vi "FPGA Main NoStartEnc.vi"() -> ()   [LabVIEW 2009]
uses:
  <vilib>/Platform/TimedLoop/XDataNode/XDataNode.xnode
  <vilib>/Platform/TimedLoop/XDataNode/loadlvalarms.vi
  <vilib>/Platform/TimedLoop/XDataNode/timing_clust.ctl
  <vilib>/Platform/TimedLoop/XDataNode/nitl_modes.ctl
  <vilib>/Platform/TimedLoop/XDataNode/wakeup.ctl
  <vilib>/eio/EIONode/EIONode.xnode
  <vilib>/rvi/eio/nirviEIOImplementation/nirviEIOImplementation.xnode
  <vilib>/rvi/eio/common/nirviEmuTemplateMethod_noerrors.vi
  <vilib>/rvi/eio/common/nirviEmuClasses.ctl
  <vilib>/Platform/TimedLoop/XDataNode/XDNodeRunTimeDep.lvlib
  <vilib>/NI VeriStand/FPGA/NI_VS FPGA Support.lvlib
panel:
  out "Travel dT (Ticks)":u32
  out "Pitch dT (Ticks)":u32
  out "Elevation dT (Ticks)":u32
  out "Travel Set High":u32
  in  "Clock Divider":u16=500
  out "Reset?":bool
  out "Travel Velocity":i32
  out "Travel Position":i32
  out "ENC 2 In Vel/Acc Update":bool
  out "Pitch Velocity":i32
  out "Pitch Position":i32
  out "ENC 1 In Vel/Acc Update":bool
  out "Elevation Velocity":i32
  out "Elevation Position":i32
  out "ENC 0 In Vel/Acc Update":bool
  in  "ENC In Clock":bool=TRUE
  in  "Fan High Time 2":u32
  in  "Fan High Time 1":u32
  out "Elevation Set High":u32
  in  "PWM Period (ticks)":u32=100000
  # "PWM In"
  # "Configuration"
  # "Internal Controls"
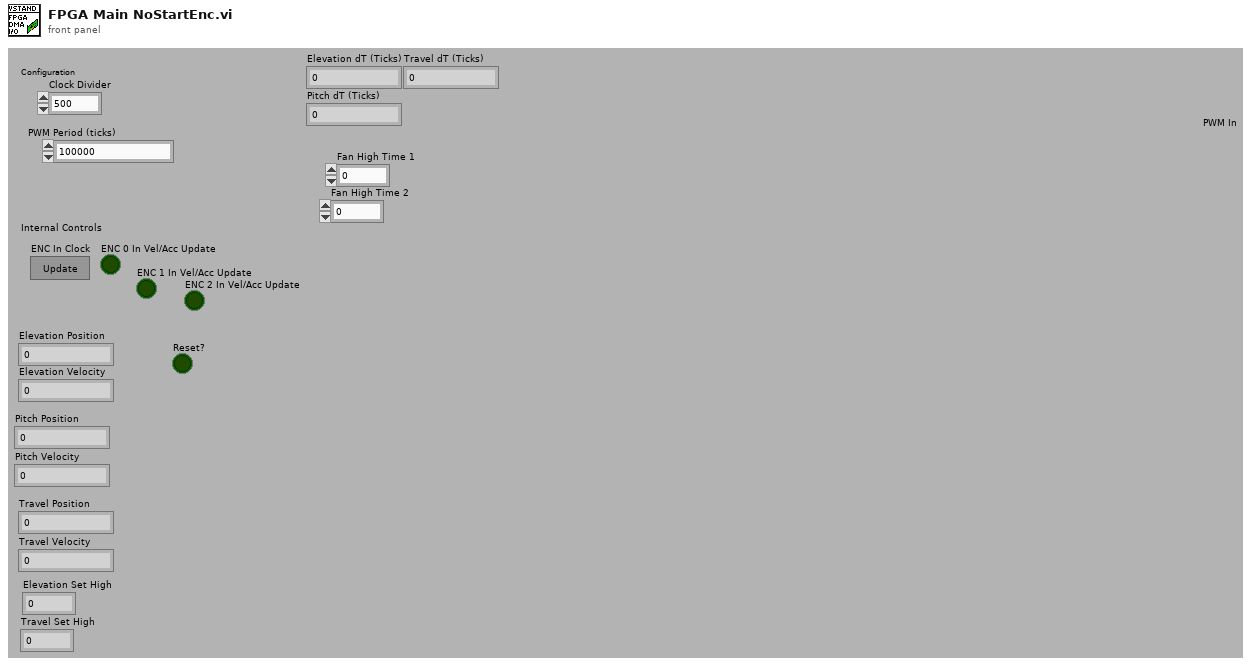
[diagram p1: front panel]
types:
  T1 = typedef "XDNodeRunTimeDep.lvlib/timing_clust.ctl" = cluster{"Expected End [f-1]":u64, "Actual End [f-1]":u64, "Finished Late? [f-1]":bool, "Expected End [i-1]":u64, "Actual End [i-1]":u64, "Finished Late? [i-1]":bool, "Expected Start [i]":u64, "Actual Start [i]":u64, "Expected Start [f]":u64, "Actual Start [f]":u64, "Source Name":string, "Structure Name":string, "Period":i64, "Deadline":i64, "Offset":i64, "Start":i64, "Priority":i32, "Timeout":i32, "Mode":T2, "Wakeup Reason":T3, "Error":errorcluster, "Source Type":string, "Secondary Source Type":string, "Global End Time":u64, "Global Start Time":u64, "Frame Duration":u64, "Iteration Duration":u64, "Assigned CPU":i32, "I/O Scan Engine Mode":u32}
  T2 = typedef "XDNodeRunTimeDep.lvlib/nitl_modes.ctl" = enum32{"No Change", "Process missed periods, maintain original phase", "Discard missed periods, maintain original phase", "Process missed periods, ignore original phase", "Discard missed periods, ignore original phase"}
  T3 = typedef "XDNodeRunTimeDep.lvlib/wakeup.ctl" = enum32{"Normal", "Aborted", "Asynchronous wakeup", "Timing source error", "Timed loop error", "Timeout"}
  T4 = typedef "nirviEmuClasses.ctl" = enum16{"IO Read", "IO Write", "Method", "Property Read", "Property Write"}
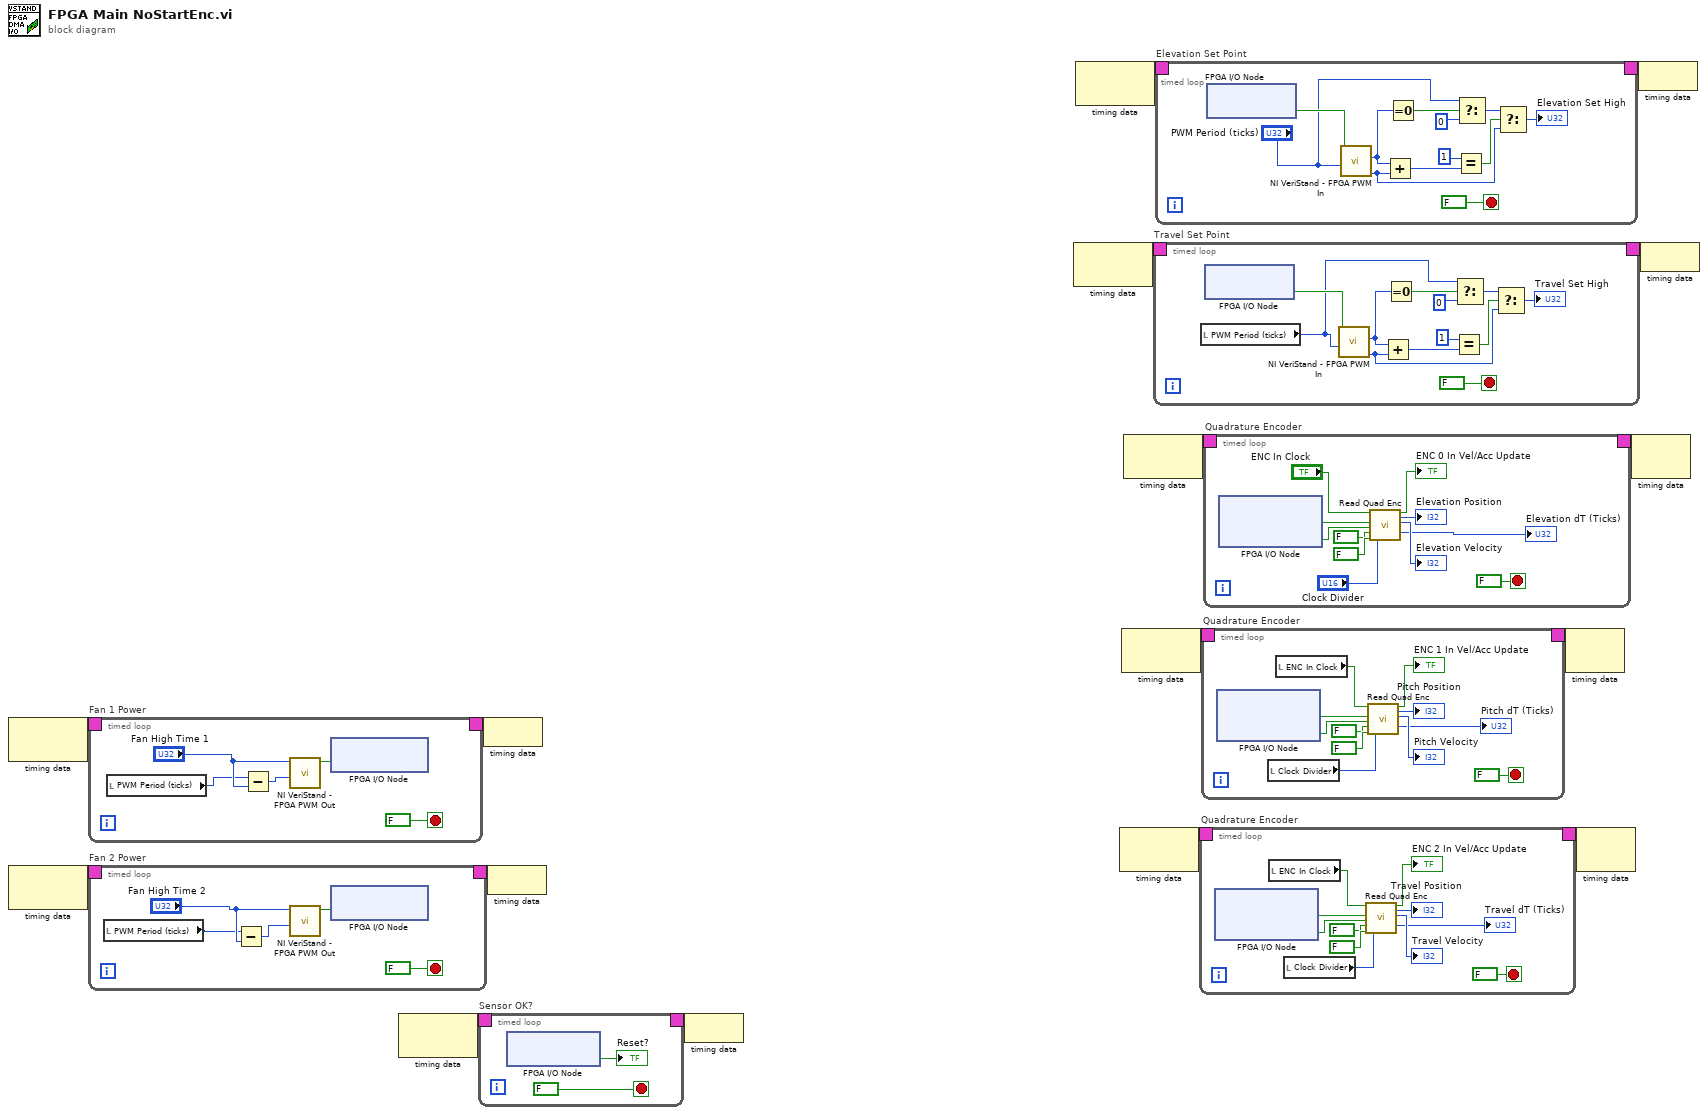
[diagram p0: block diagram]
diagram:
  n1 = node-c288() -> (w16:T1)  [unwired: 1 in]
  n2 = node-c288() -> (w14:T1)  [unwired: 1 in]
  n3 = timed-loop "Fan 1 Power" {
    timing: w16 -> [_]
    timing-out: [_] -> w15
    stop <- FALSE stop-if-true
    n4 = local read "PWM Period (ticks)"() -> (w17:u32)
    n5 = Subtract(x=w17, y="Fan High Time 1") -> (x-y=w19:u32)
    n6 = call <vilib>:"NI VeriStand - FPGA PWM Out.vi"("_Low Time"=w19, "_High Time"="Fan High Time 1") -> ("Output"=w20:bool)  [unwired: 9 in]
    n7 = xnode "FPGA I/O Node"("PWM 2 Out"=w20) -> ()  [unwired: 1 in, 1 out]
  }
  n8 = timed-loop "Fan 2 Power" {
    timing: w14 -> [_]
    timing-out: [_] -> w13
    stop <- FALSE stop-if-true
    n9 = local read "PWM Period (ticks)"() -> (w35:u32)
    n10 = Subtract(x=w35, y="Fan High Time 2") -> (x-y=w36:u32)
    n11 = call <vilib>:"NI VeriStand - FPGA PWM Out.vi"("_Low Time"=w36, "_High Time"="Fan High Time 2") -> ("Output"=w38:bool)  [unwired: 9 in]
    n12 = xnode "FPGA I/O Node"("PWM 3 Out"=w38) -> ()  [unwired: 1 in, 1 out]
  }
  n13 = node-c288() -> (w12:T1)  [unwired: 1 in]
  n14 = timed-loop "Sensor OK?" {
    timing: w12 -> [_]
    timing-out: [_] -> w11
    stop <- FALSE stop-if-true
    n15 = xnode "FPGA I/O Node"() -> ("Sensor OK"=→"Reset?":bool)  [unwired: 1 in, 1 out]
  }
  n16 = node-c288(w15) -> ()
  n17 = node-c288(w13) -> ()
  n18 = node-c288(w11) -> ()
  n19 = node-c288() -> (w2:T1)  [unwired: 1 in]
  n20 = node-c288() -> (w10:T1)  [unwired: 1 in]
  n21 = node-c288() -> (w4:T1)  [unwired: 1 in]
  n22 = node-c288() -> (w6:T1)  [unwired: 1 in]
  n23 = node-c288() -> (w8:T1)  [unwired: 1 in]
  n24 = timed-loop "Travel Set Point" {
    timing: w2 -> [_]
    timing-out: [_] -> w1
    stop <- FALSE stop-if-true
    n25 = local read "PWM Period (ticks)"() -> (w76:u32)
    n26 = xnode "FPGA I/O Node"() -> ("PWM 1 In"=w86:bool)  [unwired: 1 in, 1 out]
    n27 = call <vilib>:"NI VeriStand - FPGA PWM In.vi"("Time Out"=w76, "Value"=w86) -> ("High time"=w82:u32, "Low Time"=w80:u32)  [unwired: 8 in]
    n28 = Add(x=w80, y=w82) -> (x+y=w85:u32)
    n29 = Equal To 0?(x=w80) -> (x = 0?=w81:bool)
    n30 = Equal?(x=u32 1, y=w85) -> (x = y?=w83:bool)
    n31 = Select(t=w76, s=w81, f=u32 0) -> (s? t:f=w78:u32)
    n32 = Select(t=w78, s=w83, f=w82) -> (s? t:f=→"Travel Set High":u32)
  }
  n33 = timed-loop "Elevation Set Point" {
    timing: w10 -> [_]
    timing-out: [_] -> w9
    stop <- FALSE stop-if-true
    n34 = xnode "FPGA I/O Node"() -> ("PWM 0 In"=w119:bool)  [unwired: 1 in, 1 out]
    n35 = call <vilib>:"NI VeriStand - FPGA PWM In.vi"("Time Out"="PWM Period (ticks)", "Value"=w119) -> ("High time"=w115:u32, "Low Time"=w113:u32)  [unwired: 8 in]
    n36 = Add(x=w113, y=w115) -> (x+y=w118:u32)
    n37 = Equal To 0?(x=w113) -> (x = 0?=w114:bool)
    n38 = Equal?(x=u32 1, y=w118) -> (x = y?=w116:bool)
    n39 = Select(t="PWM Period (ticks)", s=w114, f=u32 0) -> (s? t:f=w111:u32)
    n40 = Select(t=w111, s=w116, f=w115) -> (s? t:f=→"Elevation Set High":u32)
  }
  n41 = timed-loop "Quadrature Encoder" {
    timing: w4 -> [_]
    timing-out: [_] -> w3
    stop <- FALSE ("stop") stop-if-true
    n42 = xnode "FPGA I/O Node"() -> ("ENC 2 A+ In"=w147:bool, "ENC 2 B+ In"=w146:bool)  [unwired: 2 in, 2 out]
    n43 = local read "ENC In Clock"() -> (w144:bool)
    n44 = local read "Clock Divider"() -> (w143:u16)
    n45 = call "Read Quad Enc.vi"("Clock"=w144, "A"=w147, "B"=w146, "Z"=FALSE, "Polarity"=FALSE, "Clock Divider"=w143) -> ("Vel/Acc Update"=→"ENC 2 In Vel/Acc Update":bool, "Position (Counts)"=→"Travel Position":i32, "Velocity (Counts/Interval)"=→"Travel Velocity":i32, "dT (Ticks)"=→"Travel dT (Ticks)":u32)  [unwired: 2 in, 8 out]
  }
  n46 = timed-loop "Quadrature Encoder" {
    timing: w6 -> [_]
    timing-out: [_] -> w5
    stop <- FALSE ("stop") stop-if-true
    n47 = xnode "FPGA I/O Node"() -> ("ENC 1 A+ In"=w198:bool, "ENC 1 B+ In"=w197:bool)  [unwired: 2 in, 2 out]
    n48 = local read "Clock Divider"() -> (w194:u16)
    n49 = local read "ENC In Clock"() -> (w195:bool)
    n50 = call "Read Quad Enc.vi"("Clock"=w195, "A"=w198, "B"=w197, "Z"=FALSE, "Polarity"=FALSE, "Clock Divider"=w194) -> ("Vel/Acc Update"=→"ENC 1 In Vel/Acc Update":bool, "Position (Counts)"=→"Pitch Position":i32, "Velocity (Counts/Interval)"=→"Pitch Velocity":i32, "dT (Ticks)"=→"Pitch dT (Ticks)":u32)  [unwired: 2 in, 8 out]
  }
  n51 = timed-loop "Quadrature Encoder" {
    timing: w8 -> [_]
    timing-out: [_] -> w7
    stop <- FALSE ("stop") stop-if-true
    n52 = xnode "FPGA I/O Node"() -> ("ENC 0 A+ In"=w249:bool, "ENC 0 B+ In"=w248:bool)  [unwired: 2 in, 2 out]
    n53 = call "Read Quad Enc.vi"("Clock"="ENC In Clock", "A"=w249, "B"=w248, "Z"=FALSE, "Polarity"=FALSE, "Clock Divider"="Clock Divider") -> ("Vel/Acc Update"=→"ENC 0 In Vel/Acc Update":bool, "Position (Counts)"=→"Elevation Position":i32, "Velocity (Counts/Interval)"=→"Elevation Velocity":i32, "dT (Ticks)"=→"Elevation dT (Ticks)":u32)  [unwired: 2 in, 8 out]
  }
  n54 = node-c288(w5) -> ()  [unwired: 1 out]
  n55 = node-c288(w3) -> ()  [unwired: 1 out]
  n56 = node-c288(w7) -> ()  [unwired: 1 out]
  n57 = node-c288(w9) -> ()
  n58 = node-c288(w1) -> ()
